vi "Make New Worker.vi"(6 "Selected Actions":T1, 8 "New Project?":bool, 9 "Add to Project (None)":refnum<vi>, 11 "New Worker Name":string) -> (0 "error out":errorcluster)   [LabVIEW 2022 SP3, in "FlexBlocks Support.lvlib"]
uses:
  FlexBlocks Support.lvlib
  Action Selections.ctl
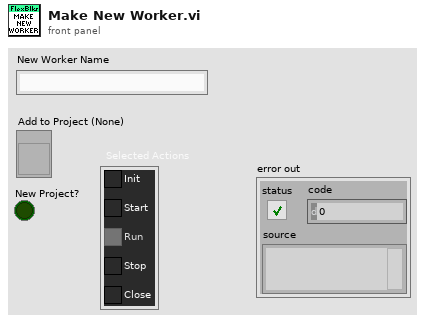
[diagram p1: front panel]
types:
  T1 = typedef "FlexBlocks Support.lvlib/Action Selections.ctl" = cluster{"Init":bool, "Start":bool, "Run":bool, "Stop":bool, "Close":bool}
  T2 = typedef "FlexBlocks Support.lvlib/Paths.ctl" = cluster{"FlexBlocks":path, "Workers Root":path, "Specialized Editors":path, "Worker Template":path, "SM Template":path, "Read Control Value Vim":path, "Write Indicator Value Vim":path}
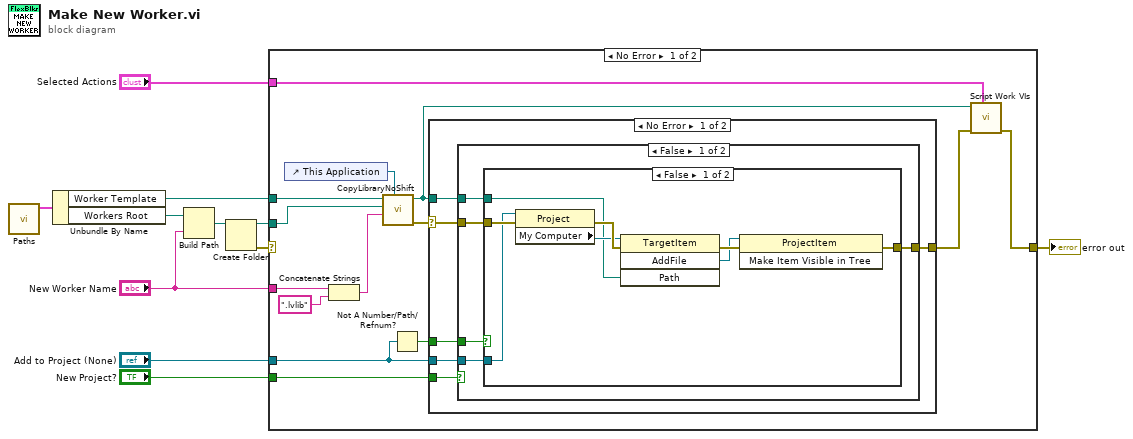
[diagram p0: block diagram]
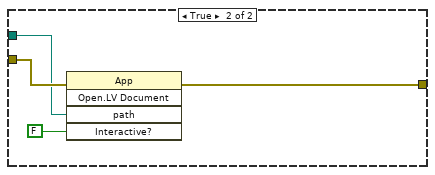
[diagram p2: hidden frame]
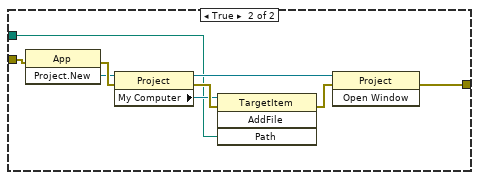
[diagram p3: hidden frame]
diagram:
  n1 = call "Paths.vi"() -> ("Paths"=w11:T2)  [unwired: 11 in]
  n2 = Unbundle By Name(w11) -> ("Worker Template"=w6:path, "Workers Root"=w10:path)
  n3 = Build Path(base path=w10, name or relative path="New Worker Name") -> (appended path=w9:path)
  n4 = Create Folder(path (use dialog)=w9) -> (created path=w7:path, error out=w8:errorcluster)  [unwired: 2 in, 1 out]
  n5 = case shown="No Error" w8 {
    selector: w8 -> [_ w59]
    tunnel: w7 -> [w24 _]
    tunnel: w6 -> [w25 _]
    tunnel: "New Worker Name" -> [w22 _]
    tunnel: "Add to Project (None)" -> [w17 _]
    tunnel: "New Project?" -> [w18 _]
    tunnel: [w13 w59] -> w2
    tunnel: "Selected Actions" -> [w12 _]
    frame No Error {
      n6 = control-ref of="This Application"() -> (w23:refnum<vi>)
      n7 = Concatenate Strings(w22, ".lvlib" ("string")) -> (w20:string)
      n8 = call "CopyLibraryNoShift.vi"("app"=w23, "new library name"=w20, "new folder"=w24, "source library path"=w25) -> ("error out"=w19:errorcluster, "copied library path"=w15:path)  [unwired: 5 in, 1 out]
      n9 = Not A Number/Path/Refnum?(number/path/refnum=w17) -> (NaN/Path/Refnum?=w16:bool)
      n10 = case shown="No Error" w19 {
        selector: w19 -> [w29 w58]
        tunnel: w15 -> [w31 _]
        tunnel: w18 -> [w30 _]
        tunnel: w17 -> [w26 _]
        tunnel: w16 -> [w27 _]
        tunnel: [w28 w58] -> w14
        frame No Error {
          n11 = case shown="False" w30 {
            tunnel: w31 -> [w34 w50]
            tunnel: w29 -> [w33 w51]
            tunnel: [w32 w49] -> w28
            tunnel: w27 -> [w36 _]
            tunnel: w26 -> [w35 _]
            frame False {
              n12 = case shown="False" w36 {
                tunnel: w35 -> [w41 _]
                tunnel: w34 -> [w40 w46]
                tunnel: w33 -> [w42 w48]
                tunnel: [w37 w45] -> w32
                frame False {
                  n13 = property class="Project"(reference=w41, error in=w42) -> (error out=w44:errorcluster, "My Computer"=w43:refnum<vi>)  [unwired: 1 out]
                  n14 = invoke class="TargetItem" method="AddFile"(reference=w43, error in=w44, "Path"=w40) -> (error out=w39:errorcluster, "AddFile"=w38:refnum<vi>)  [unwired: 1 in, 2 out]
                  n15 = invoke class="ProjectItem" method="Make Item Visible in Tree"(reference=w38, error in=w39) -> (error out=w37:errorcluster)  [unwired: 1 in, 2 out]
                }
                frame True {
                  n16 = invoke class="App" method="Open.LV Document"(error in=w48, "path"=w46, "Interactive?"=FALSE) -> (error out=w45:errorcluster)  [unwired: 2 in, 4 out]
                }
              }
            }
            frame True {
              n17 = invoke class="App" method="Project.New"(error in=w51) -> (error out=w56:errorcluster, "Project:New"=w55:refnum<vi>)  [unwired: 2 in, 1 out]
              n18 = property class="Project"(reference=w55, error in=w56) -> (reference out=w53:refnum<vi>, error out=w57:errorcluster, "My Computer"=w54:refnum<vi>)
              n19 = invoke class="TargetItem" method="AddFile"(reference=w54, error in=w57, "Path"=w50) -> (error out=w52:errorcluster)  [unwired: 1 in, 3 out]
              n20 = invoke class="Project" method="Open Window"(reference=w53, error in=w52) -> (error out=w49:errorcluster)  [unwired: 1 in, 2 out]
            }
          }
        }
        frame Error {
        }
      }
      n21 = call "Script Work VIs.vi"("Selected Actions"=w12, "error in (no error)"=w14, "Worker Library Path"=w15) -> ("error out"=w13:errorcluster)  [unwired: 8 in]
    }
    frame Error {
    }
  }
  "error out" <- w2
